vi "Get-safe.vi"(8 "error in (no error)":errorcluster, 11 "Motor-Maxon in":refnum<class "Motor-Maxon.lvclass">) -> (0 "error out":errorcluster, 1 "Safe?":bool, 3 "Motor-Maxon out":refnum<class "Motor-Maxon.lvclass">)   [LabVIEW 2013, in "PowderDeposition.lvlib" / "Motor-Maxon.lvclass"]
uses:
  Motor-Maxon.lvclass
  Motor-Maxon.lvclass/Motor-Maxon.ctl
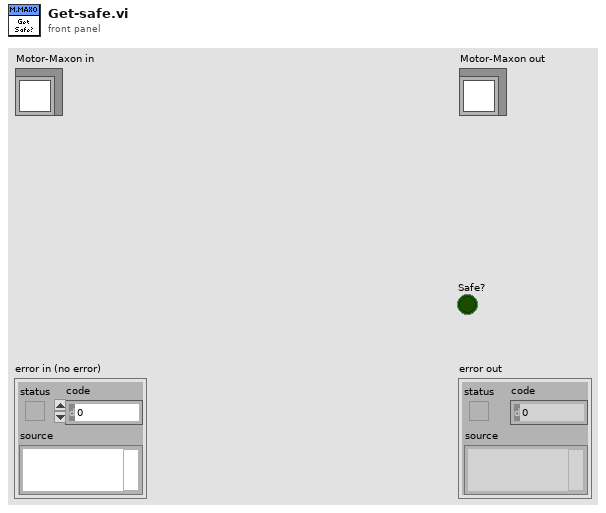
[diagram p1: front panel]
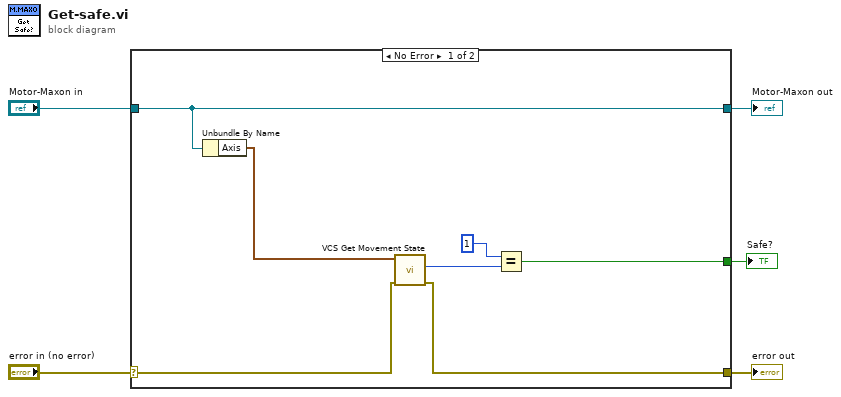
[diagram p0: block diagram]
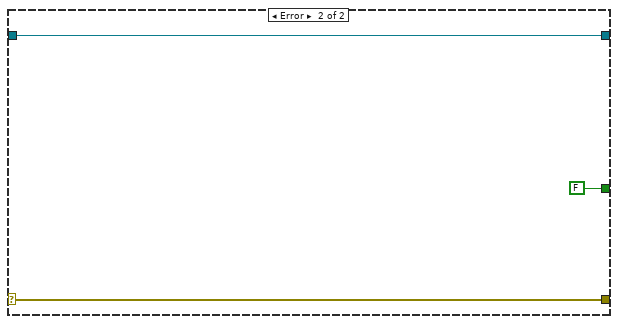
[diagram p2: hidden frame]
diagram:
  n1 = case shown="No Error" "error in (no error)" {
    selector: "error in (no error)" -> [w7 w15]
    tunnel: [w6 w15] -> w4
    tunnel: [w11 w14] -> w2
    tunnel: "Motor-Maxon in" -> [w11 w14]
    tunnel: [w8 FALSE] -> w1
    frame No Error {
      n2 = Unbundle By Name(w11) -> ("Axis"=w10:cluster{"keyHandle":u32, "nodeID":u16})
      n3 = call <instrlib>:"VCS Get Movement State.vi"("error in (no error)"=w7, "axis in"=w10) -> ("error out"=w6:errorcluster, "targetReached"=w9:i32)  [unwired: 7 in, 1 out]
      n4 = Equal?(x=1, y=w9) -> (x = y?=w8:bool)
    }
    frame Error {
    }
  }
  "error out" <- w4
  "Motor-Maxon out" <- w2
  "Safe?" <- w1
